vi "Test Error Cluster.vi"(11 "Test Case In":refnum<class "Describe Variant Test.lvclass">) -> (0 "error out":errorcluster, 3 "Test Case Out":refnum<class "Describe Variant Test.lvclass">)   [LabVIEW 2020, in "Describe Variant Test.lvclass"]
uses:
  Describe Variant Test.lvclass
  C:/Program Files (x86)/National Instruments/LabVIEW 2020/vi.lib/Astemes/LUnit/Test Case.lvclass
  <vilib>/Astemes/LUnit/Test Case.lvclass/Test Case.ctl
  7c39a56f-5538-4c7e-9d72-f297bb98ba6b.vi
  <vilib>/Astemes/LUnit/Core/LUnit Test Case/Private/Append Pass Result.vi
  <vilib>/Astemes/LUnit/Core/LUnit Test Case/Private/Append Fail Result.vi
  7c39a56f-5538-4c7e-9d72-f297bb98ba6b.vi/9c5d11cd-9439-4240-a1ee-d9baace9c924.vi
  <vilib>/Astemes/LUnit/Core/LUnit Test Case/Private/Run In UI.vi
  <vilib>/Utility/error.llb/Clear Errors.vi
  source/Framework/Utilities/Utilities.lvlib
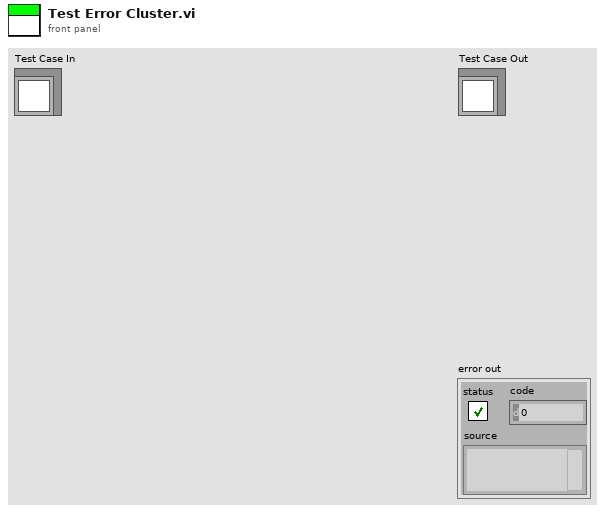
[diagram p1: front panel]
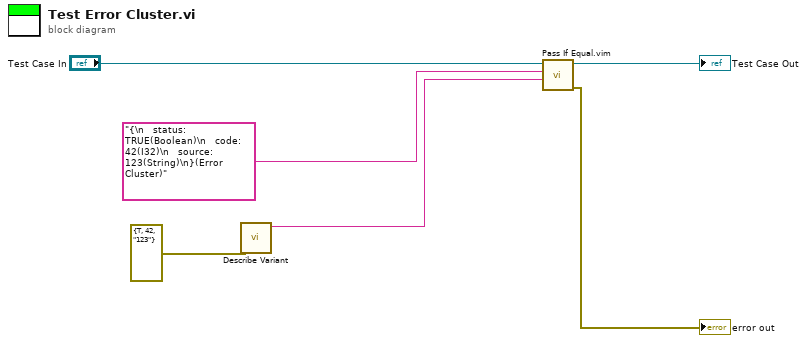
[diagram p0: block diagram]
diagram:
  n1 = call "Describe Variant.vi"("Variant"=errorcluster {"status"=TRUE, "code"=42, "source"="123"} ("error constant")) -> ("Variant Description"=w3:string)  [unwired: 8 in, 2 out]
  n2 = call "Pass If Equal.vim"("Actual"=w3, "Expected"="{\n   status: TRUE(Boolean)\n   code: 42(I32)\n   source: 123(String)\n}(Error Cluster)", "LUnit Test Case In"="Test Case In") -> ("error out"=→"error out":errorcluster, "LUnit Test Case Out"=→"Test Case Out":refnum<class "Describe Variant Test.lvclass">)  [unwired: 7 in]
